vi "Inst.Krohn-Hite-7008.handleGetCommand.vi"(8 "error in (no error)":errorcluster, 9 "Data":variant, 10 "Command in":string, 11 "Inst.Krohn-Hite-7008 in":refnum<class "Inst.Krohn-Hite-7008.lvclass">) -> (0 "error out":errorcluster, 1 "output cluster":T1={"allChannelProperties"=[{"channel"=1, "gain"=enum."10", "input"=enum."OFF", "shunt"=enum."10M", "couple"=enum."AC", "filter"=enum."OFF"}, {"channel"=2, "gain"=enum."10", "input"=enum."OFF", "shunt"=enum."10M", "couple"=enum."AC", "filter"=enum."OFF"}, {"channel"=3, "gain"=enum."10", "input"=enum."OFF", "shunt"=enum."10M", "couple"=enum."AC", "filter"=enum."OFF"}, {"channel"=4, "gain"=enum."10", "input"=enum."OFF", "shunt"=enum."10M", "couple"=enum."AC", "filter"=enum."OFF"}, {"channel"=5, "gain"=enum."10", "input"=enum."OFF", "shunt"=enum."10M", "couple"=enum."AC", "filter"=enum."OFF"}, {"channel"=6, "gain"=enum."10", "input"=enum."OFF", "shunt"=enum."10M", "couple"=enum."AC", "filter"=enum."OFF"}, {"channel"=7, "gain"=enum."10", "input"=enum."OFF", "shunt"=enum."10M", "couple"=enum."AC", "filter"=enum."OFF"}, {"channel"=7, "gain"=enum."10", "input"=enum."OFF", "shunt"=enum."10M", "couple"=enum."AC", "filter"=enum."OFF"}]} {"allChannelProperties"."channel" min=1 max=8 step=1}, 2 "Command out":string, 3 "Inst.Krohn-Hite-7008 out":refnum<class "Inst.Krohn-Hite-7008.lvclass">)   [LabVIEW 2019, in "Inst.KH7008.lvlib" / "Inst.Krohn-Hite-7008.lvclass"]
uses:
  Inst.Krohn-Hite-7008.lvclass
  Inst.Krohn-Hite-7008.lvclass/Inst.Krohn-Hite-7008.ctl
  Typedefs/getChannelRequest--Cluster.ctl
  KH7008/typedefs/channel--numeric.ctl
  a0eabf90-b4d9-4584-866f-9f1db62b2114.vi
  a0eabf90-b4d9-4584-866f-9f1db62b2114.vi/c33843f7-451f-4e2e-a4e3-fc07b03aa2e1.vi
  a0eabf90-b4d9-4584-866f-9f1db62b2114.vi/53209b5d-dba8-4aeb-859b-6a1b8073345c.vi
  <vilib>/Utility/Data Type/Get Type Information.vi
  <vilib>/JDP Science/JSONtext/JSON text to Variant.vi
  <vilib>/JDP Science/JSONtext/LVClass Serializer/JSONtext LVClass Serializer.lvclass
  KH7008/KH7008.lvlib
  KH7008/typedefs/Filter--Enum.ctl
  KH7008/typedefs/couple--Enum.ctl
  KH7008/typedefs/shunt--enum.ctl
  KH7008/typedefs/Input--Enum.ctl
  KH7008/typedefs/gain--enum.ctl
  KH7008/typedefs/channelProperties--Cluster.ctl
  KH7008/typedefs/allChannelProperties--Array.ctl
  Typedefs/getAllChannelsResponse--Cluster.ctl
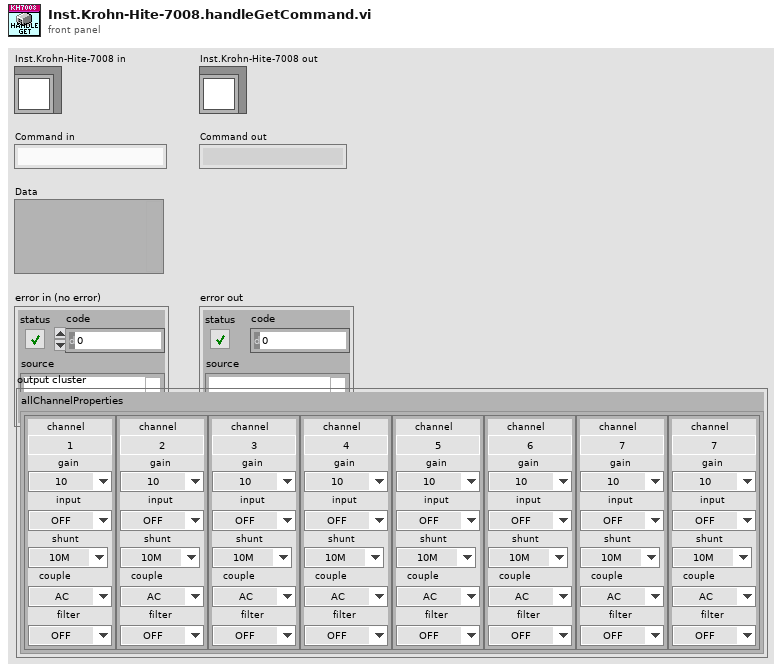
[diagram p1: front panel]
types:
  T1 = typedef "Inst.KH7008.lvlib/Inst.Krohn-Hite-7008.lvclass/getAllChannelsResponse--Cluster.ctl" = cluster{"allChannelProperties":T2}
  T2 = typedef "KH7008.lvlib/allChannelProperties--Array.ctl" = T3[]
  T3 = typedef "KH7008.lvlib/channelProperties--Cluster.ctl" = cluster{"channel":T4, "gain":T5, "input":T6, "shunt":T7, "couple":T8, "filter":T9}
  T4 = typedef "KH7008.lvlib/channel--numeric.ctl" = u16
  T5 = typedef "KH7008.lvlib/gain--enum.ctl" = enum16{"1", "10", "100", "1000"}
  T6 = typedef "KH7008.lvlib/input--enum.ctl" = enum16{"OFF", "SE+", "SE-", "DIFF"}
  T7 = typedef "KH7008.lvlib/shunt--enum.ctl" = enum16{"Open", "50", "500", "5k", "50k", "10M"}
  T8 = typedef "KH7008.lvlib/couple--enum.ctl" = enum16{"AC", "DC"}
  T9 = typedef "KH7008.lvlib/filter--enum.ctl" = enum16{"OFF", "ON"}
  T10 = typedef "Inst.KH7008.lvlib/Inst.Krohn-Hite-7008.lvclass/getChannelRequest--Cluster.ctl" = cluster{"channel":T4}
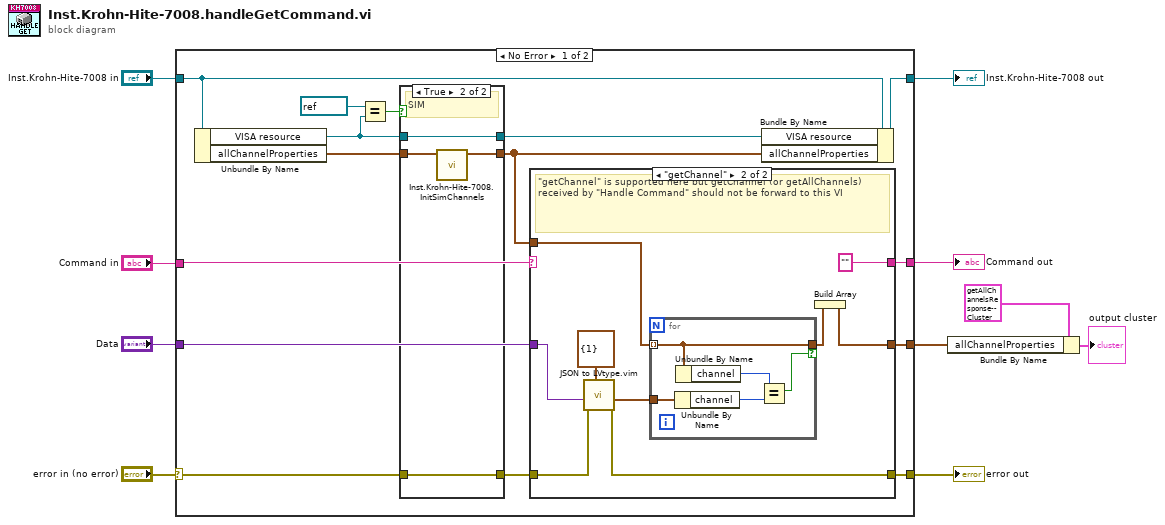
[diagram p0: block diagram]
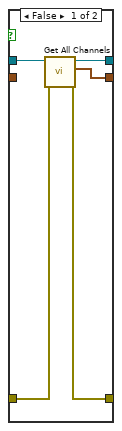
[diagram p2: hidden frame]
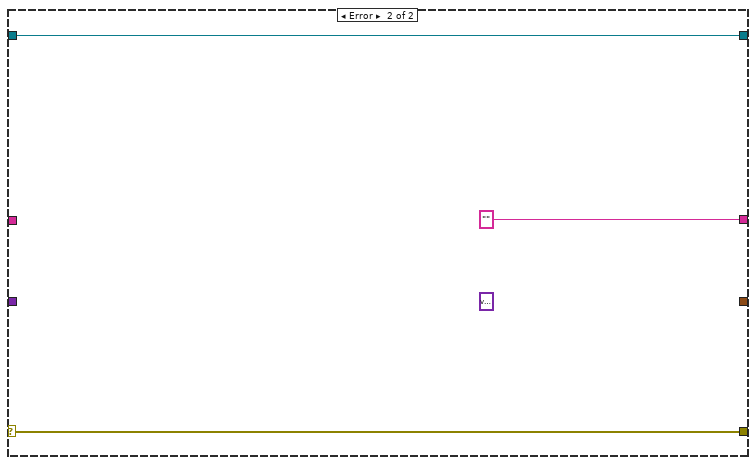
[diagram p4: hidden frame]
diagram:
  n1 = case shown="No Error" "error in (no error)" {
    selector: "error in (no error)" -> [w25 w54]
    tunnel: [w24 w54] -> w9
    tunnel: [w19 w53] -> w8
    tunnel: "Inst.Krohn-Hite-7008 in" -> [w21 w53]
    tunnel: [w16 "" ("Command")] -> w6
    tunnel: "Command in" -> [w23 _]
    tunnel: "Data" -> [w20 _]
    tunnel: [w11 _] -> w3
    frame No Error {
      n2 = Unbundle By Name(w21) -> ("VISA resource"=w12:refnum<visa-resource-name>, "allChannelProperties"=w17:T2)
      n3 = Equal?(x=refnum<visa-resource-name> "sim" ("y"), y=w12) -> (x = y?=w14:bool)
      n4 = case shown="True" w14 {
        tunnel: [w30 w34] -> w22
        tunnel: w25 -> [w29 w33]
        tunnel: [w28 w32] -> w18
        tunnel: [w27 w33] -> w15
        tunnel: w12 -> [w26 w34]
        tunnel: w17 -> [_ w31]
        frame False {
          n5 = call "Get All Channels.vi"("error in (no error)"=w29, "VISA Refnum in"=w26) -> ("error out"=w27:errorcluster, "allChannelProperties"=w28:T2, "VISA Refnum out"=w30:refnum<visa-resource-name>)  [unwired: 7 in]
        }
        frame True {
          # "SIM"
          n6 = call "Inst.Krohn-Hite-7008.InitSimChannels.vi"("allChannelProperties"=w31) -> ("allChannelProperties"=w32:T2)  [unwired: 10 in]
        }
      }
      n7 = case shown="\"getChannel\"" w23 {
        selector: w23 -> [w36 _]
        tunnel: w18 -> [w35 w42]
        tunnel: w20 -> [_ w45]
        tunnel: w15 -> [w37 w44]
        tunnel: [w37 w40] -> w24
        tunnel: [w36 ""] -> w16
        tunnel: [w35 w38] -> w11
        frame "getAllChannels", Default {
        }
        frame "getChannel" {
          # "\"getChannel\" is supported here but getChannel (or getAllChannels) received by \"Handle Command\" should not be forward to this VI"
          n8 = call "JSON to LVtype.vim"("type"=T10 {"channel"=1} ("getChannelRequest"), "error in (no error)"=w44, "JSON Data in"=w45) -> ("error out"=w40:errorcluster, "Data out"=w43:T10)  [unwired: 7 in]
          n9 = for {
            tunnel: w42 -> [w50] mode=indexing
            tunnel: [w50] -> w39 if=w49
            tunnel: w43 -> [w48]
            n10 = Unbundle By Name(w48) -> ("channel"=w47:T4)
            n11 = Unbundle By Name(w50) -> ("channel"=w51:T4)
            n12 = Equal?(x=w51, y=w47) -> (x = y?=w49:bool)
          }
          n13 = Build Array(w39) -> (w38:T3[])
        }
      }
      n14 = Bundle By Name(cluster=w21, "VISA resource"=w22, "allChannelProperties"=w18) -> (w19:refnum<class "Inst.Krohn-Hite-7008.lvclass">)
    }
    frame Error {
      (unwired) variant ("Variant")
    }
  }
  "error out" <- w9
  "Inst.Krohn-Hite-7008 out" <- w8
  "Command out" <- w6
  n15 = Bundle By Name(cluster=T1 {"allChannelProperties"=[{"channel"=1, "gain"=enum."10", "input"=enum."OFF", "shunt"=enum."10M", "couple"=enum."AC", "filter"=enum."OFF"}, {"channel"=2, "gain"=enum."10", "input"=enum."OFF", "shunt"=enum."10M", "couple"=enum."AC", "filter"=enum."OFF"}, {"channel"=3, "gain"=enum."10", "input"=enum."OFF", "shunt"=enum."10M", "couple"=enum."AC", "filter"=enum."OFF"}, {"channel"=4, "gain"=enum."10", "input"=enum."OFF", "shunt"=enum."10M", "couple"=enum."AC", "filter"=enum."OFF"}, {"channel"=5, "gain"=enum."10", "input"=enum."OFF", "shunt"=enum."10M", "couple"=enum."AC", "filter"=enum."OFF"}, {"channel"=6, "gain"=enum."10", "input"=enum."OFF", "shunt"=enum."10M", "couple"=enum."AC", "filter"=enum."OFF"}, {"channel"=7, "gain"=enum."10", "input"=enum."OFF", "shunt"=enum."10M", "couple"=enum."AC", "filter"=enum."OFF"}, {"channel"=7, "gain"=enum."10", "input"=enum."OFF", "shunt"=enum."10M", "couple"=enum."AC", "filter"=enum."OFF"}]} ("getAllChannelsResponse"), "allChannelProperties"=w3) -> (→"output cluster":T1)
